vi "FormatVoltageArray.vi"(11 "Array in":dbl[](array[numeric])) -> (0 "Mirror Array":u16[](array[numeric]), 3 "Voltage Map":dbl[][](array[numeric]))   [LabVIEW 2014]
uses:
  <vilib>/Analysis/baseanly.llb/Mean (DBL).vi
  <vilib>/Analysis/NI_AALBase.lvlib
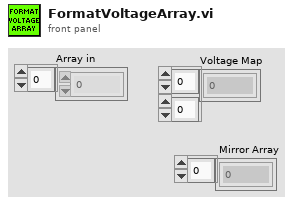
[diagram p1: front panel]
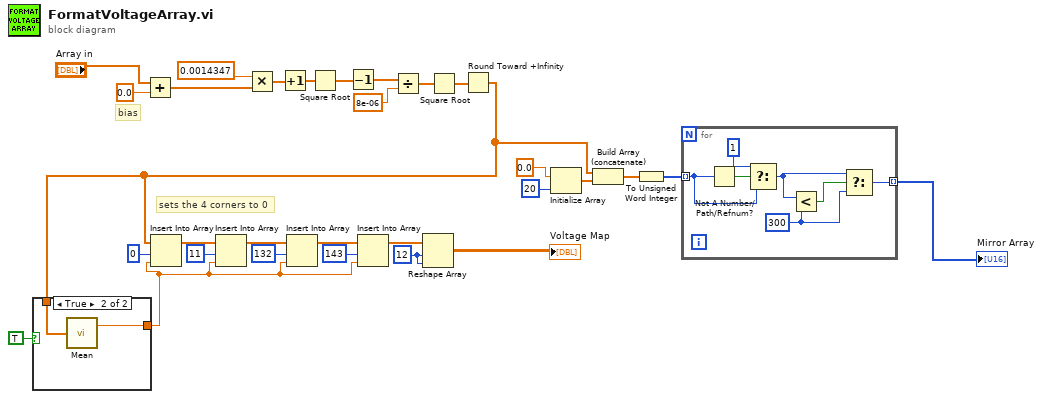
[diagram p0: block diagram]
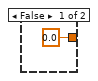
[diagram p2: hidden frame]
diagram:
  w22 = 12 ("dimension size")
  # "bias"
  # "sets the 4 corners to 0"
  n1 = Add(x="Array in", y=0.0) -> (x+y=w7:dbl[])
  n2 = Multiply(x=0.0014347, y=w7) -> (x*y=w6:dbl[])
  n3 = Increment(x=w6) -> (x+1=w5:dbl[])
  n4 = Square Root(x=w5) -> (sqrt(x)=w4:dbl[])
  n5 = Decrement(x=w4) -> (x-1=w2:dbl[])
  n6 = Divide(x=w2, y=8e-06) -> (x/y=w1:dbl[])
  n7 = Square Root(x=w1) -> (sqrt(x)=w19:dbl[])
  n8 = Round Toward +Infinity(x=w19) -> (ceil(x): smallest int >= x=w12:dbl[])
  n9 = case shown="True" TRUE {
    tunnel: w12 -> [_ w33]
    tunnel: [0.0 ("mean") w32] -> w11
    frame False {
    }
    frame True {
      n10 = call-poly <vilib>:"Mean.vi"("X"=w33) -> ("mean"=w32:dbl)  [unwired: 1 out]
    }
  }
  n11 = Insert Into Array(array=w12, index=0, new element=w11) -> (w27:dbl[])
  n12 = Insert Into Array(array=w27, index=11, new element=w11) -> (w25:dbl[])
  n13 = Insert Into Array(array=w25, index=132, new element=w11) -> (w23:dbl[])
  n14 = Insert Into Array(array=w23, index=143, new element=w11) -> (w21:dbl[])
  n15 = Reshape Array "Reshape Array"(w21, w22, w22) -> (→"Voltage Map":dbl[][])
  n16 = Initialize Array(0.0 ("element"), 20 ("dimension size")) -> (w18:dbl[])
  n17 = Build Array (concatenate)(w12, w18) -> (w15:dbl[])
  n18 = To Unsigned Word Integer(number=w15) -> (unsigned 16bit integer=w14:u16[])
  n19 = for {
    tunnel: w14 -> [w39] mode=indexing
    tunnel: [w34] -> w13 mode=indexing
    w35 = u16 300 ("y")
    n20 = Not A Number/Path/Refnum?(number/path/refnum=w39) -> (NaN/Path/Refnum?=w40:bool)
    n21 = Select(t=u16 1, s=w40, f=w39) -> (s? t:f=w36:u16)
    n22 = Less?(x=w36, y=w35) -> (x < y?=w37:bool)
    n23 = Select(t=w36, s=w37, f=w35) -> (s? t:f=w34:u16)
  }
  "Mirror Array" <- w13
